vi "XYStage.GetProtectedEvents.vi"(8 "error in (no error)":errorcluster, 11 "XYStage":refnum<class "XYStage.lvclass">) -> (0 "error out":errorcluster, 2 "Protected Events":T1, 3 "XYStage out":refnum<class "XYStage.lvclass">)   [LabVIEW 2019, in "XYStage.lvclass"]
doc: "---------------------------------------------------------------\nJKI State Machine Objects™\nhttp://jki.net/state-machine-objects/\nCopyright (C) 2005-2015, JKI <info@jki.net>\nALL RIGHTS RESERVEDJKI State Machine Objects (SMO) 1.0.0.5\nJKI - JKI\nCopyright (c) 2016, JKI"
uses:
  XYStage.lvclass
  Typedefs/API Inputs--Cluster.ctl
  Typedefs/ProtectedEvents--Cluster.ctl
panel:
  # "For instructions on how to use the JKI State Machine Objects, examples and video tutorials, visit:\nhttp://jki.net/state-machine-objects/\n\nJKI State Machine Objects™\nhttp://jki.net/state-machine-objects/\nCopyright (C) 2005-2015, JKI <info@jki.net>\nALL RIGHTS RESERVED"
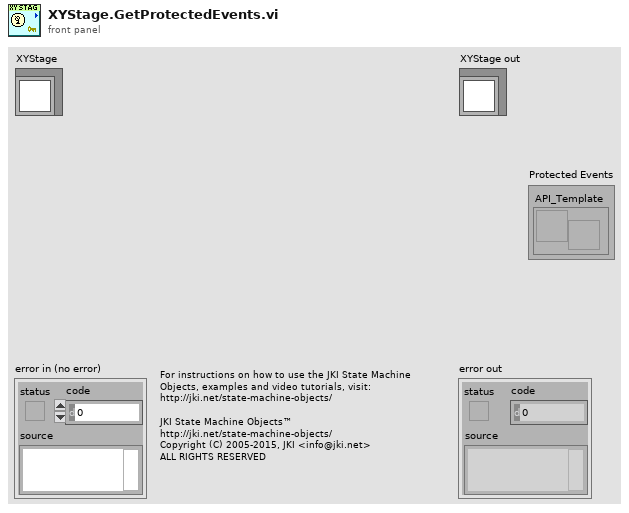
[diagram p1: front panel]
types:
  T1 = typedef "XYStage.lvclass/ProtectedEvents--Cluster.ctl" = cluster{"API_Template":refnum<user-event>}
  T2 = typedef "XYStage.lvclass/PrivateData--Ref.ctl" = refnum<data-value>
  T3 = typedef "XYStage.lvclass/PrivateData--Cluster.ctl" = cluster{"Dependencies":T4, "Public Events":T5, "Protected Events":T1, "Private Events":T6, "Configuration":T7, "Target":T8, "Move Parameters":T11}
  T4 = typedef "XYStage.lvclass/Dependencies--Cluster.ctl" = cluster{"Positions":refnum<class "SMO.Dictionary.Variant.lvclass">}
  T5 = typedef "XYStage.lvclass/PublicEvents--Cluster.ctl" = cluster{"MoveComplete":refnum<user-event>, "NewPosition":refnum<user-event>, "UpdatedNamedPosition":refnum<user-event>, "MoveStarted":refnum<user-event>}
  T6 = typedef "XYStage.lvclass/PrivateEvents--Cluster.ctl" = cluster{"MoveAbsolute":refnum<user-event>, "MoveRelative":refnum<user-event>, "MoveToNamedPosition":refnum<user-event>, "StorePosition":refnum<user-event>, "Home":refnum<user-event>}
  T7 = typedef "XYStage.lvclass/Configuration--Cluster.ctl" = cluster{"Real-World Units":string, "Counts per Unit":dbl}
  T8 = typedef "XYStage.lvclass/TargetPositions--Cluster.ctl" = cluster{"Coords":T9, "Counts":T10}
  T9 = typedef "XYStage.lvclass/(real)Coords--Cluster.ctl" = cluster{"X":dbl, "Y":dbl}
  T10 = typedef "XYStage.lvclass/(counts)Coords--Cluster.ctl" = cluster{"X":i32, "Y":i32}
  T11 = typedef "XYStage.lvclass/MoveParameters--Cluster.ctl" = cluster{"Velocity (units/s)":dbl, "Acceleration (units/s^2)":dbl}
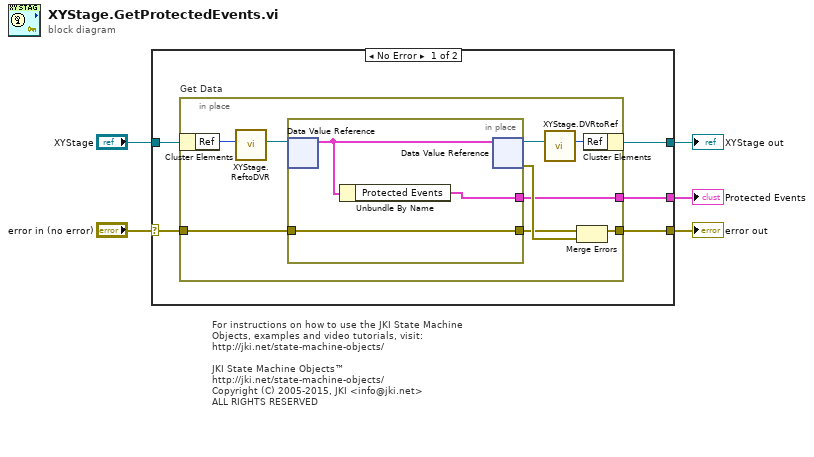
[diagram p0: block diagram]
diagram:
  # "For instructions on how to use the JKI State Machine Objects, examples and video tutorials, visit:\nhttp://jki.net/state-machine-objects/\n\nJKI State Machine Objects™\nhttp://jki.net/state-machine-objects/\nCopyright (C) 2005-2015, JKI <info@jki.net>\nALL RIGHTS RESERVED"
  n1 = case shown="No Error" "error in (no error)" {
    selector: "error in (no error)" -> [w9 w23]
    tunnel: "XYStage" -> [w10 w24]
    tunnel: [w8 w23] -> w4
    tunnel: [w7 w24] -> w3
    tunnel: [w6 _] -> w1
    frame No Error {
      n2 = in-place "Get Data" {
        in-place-border: w9 -> [w19]
        in-place-border: [w16] -> w8
        in-place-border: [w15] -> w6
        n3 = in-place-cluster #1(w10) -> ("Ref"=w12:u32)
        n4 = call "XYStage.ReftoDVR.vi"("Ref"=w12) -> ("Ref"=w11:T2)  [unwired: 10 in]
        n5 = in-place {
          in-place-border: w19 -> [w22]
          in-place-border: [w22] -> w17
          in-place-border: [w21] -> w15
          n6 = in-place-dvr #2(w11) -> (w20:T3)  [unwired: 1 out]
          n7 = Unbundle By Name(w20) -> ("Protected Events"=w21:T1)
          n8 = in-place-dvr #2(w20) -> (w14:T2, w18:errorcluster)
        }
        n9 = call "XYStage.DVRtoRef.vi"("Ref"=w14) -> ("Ref"=w13:u32)  [unwired: 10 in]
        n10 = Merge Errors(w17, w18) -> (w16:errorcluster)
        n11 = in-place-cluster #1("Ref"=w13) -> (w7:refnum<class "XYStage.lvclass">)
      }
    }
    frame Error {
    }
  }
  "error out" <- w4
  "XYStage out" <- w3
  "Protected Events" <- w1
